vi "BotSpeak_AskDevice.vi"(3 "Bot Settings":T2) -> (1 "Bot Settings out":T2)   [LabVIEW 2012]
uses:
  <userlib>/BotSpeak/VIs/Direct/BotSpeak_Control.ctl
  <vilib>/Platform/browser.llb/Open URL in Default Browser (string).vi
  <userlib>/BotSpeak/VIs/SubVIs/BotSpeak_Globals.vi
panel:
  out "Finished":bool
  in  "View":enum32{"Normal", "Testing"}(tab)
  out "Help":string
  in  "Hardware":u16(ring) items=["Arduino Uno", "BeagleBone Serial", "BeagleBone", "Console Only", "EvalRIO", "Galileo", "Launchpad", "PICAXE 80M", "Raspberry Pi", "Thymio"]
  in  "Done":bool
  in  "Cancel":bool
  in  "Connection":T1(tab)
  in  "IP Address":string(combo)
  in  "VISA":u16(ring) items=["ASRL7  (COM7 - Galileo)", "ASRL4  (COM4 - Intel(R) Active Management Technology - SOL)", "ASRL3  (COM3)"]
  in  "Test":bool
  in  "Goto URL":bool
  out "URL":string
  out "Status":string
  out "firmware":dbl
  in  "Back":bool
  out "List":string[](array[string])
  # "For More Help:"
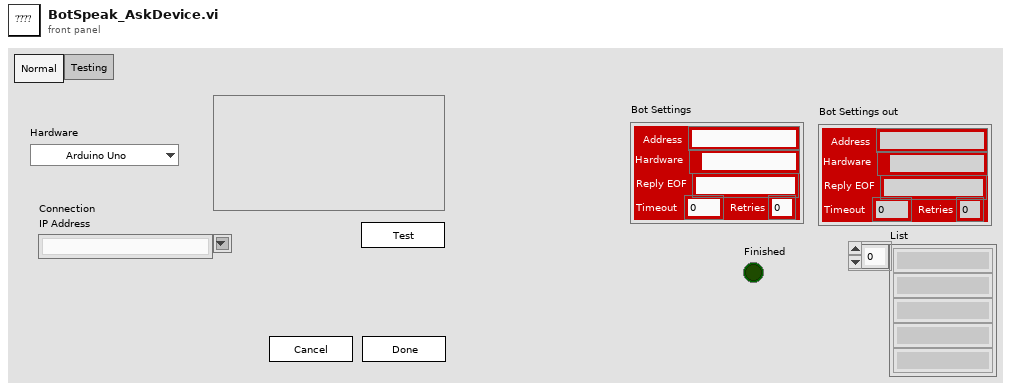
[diagram p1: front panel]
types:
  T1 = enum32{"TCPIP", "Serial", "Undefined", "Console"}
  T2 = typedef "BotSpeak_Control.ctl" = cluster{"Address":string, "Reply EOF":string, "Hardware":path, "Retries":i8, "Timeout":i32}
  T3 = typedef "BotSpeak.HardwareSpecs.ctl" = cluster{"Hardware Name":string, "Hardware URL":string, "ComType":enum16{"Undefined", "Serial", "TCPIP", "Console"}, "TCP Port":i32, "DefaultAddress":string, "Retries":i32, "Translate":enum16{"None", "Tiny", "URAPI"}, "MaxScriptSize":i32, "MaxVarNumber":i32, "StartupWait":i32, "Patience":i32, "Startup Patience":i32, "Hardware Help":string, "Com Protocol":string, "Translator":cluster{"BotSpeak CMD":string, "CMD out":string}[], "Init Code":string, "Variable Format":enum16{"INT", "FLOAT", "FIXED"}}
  T4 = enum16{"Undefined", "Serial", "TCPIP", "Console"}
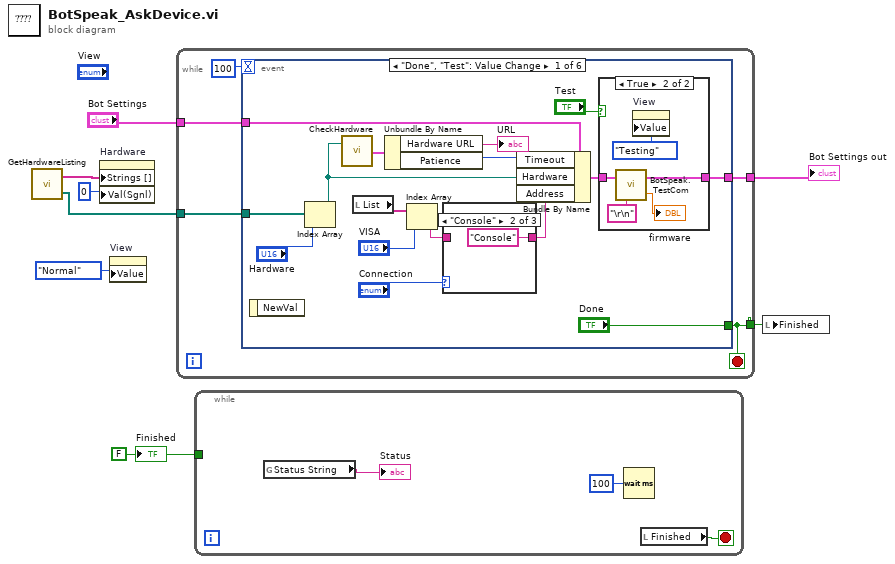
[diagram p0: block diagram]
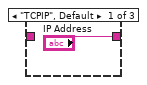
[diagram p2: hidden frame]
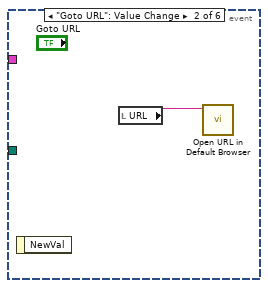
[diagram p5: hidden frame]
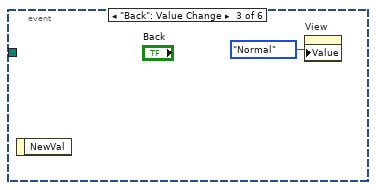
[diagram p6: hidden frame]
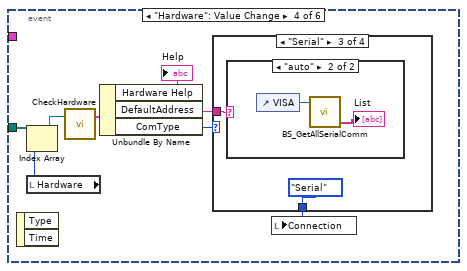
[diagram p7: hidden frame]
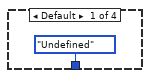
[diagram p8: hidden frame]
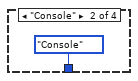
[diagram p9: hidden frame]
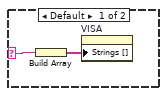
[diagram p10: hidden frame]
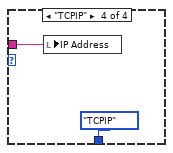
[diagram p11: hidden frame]
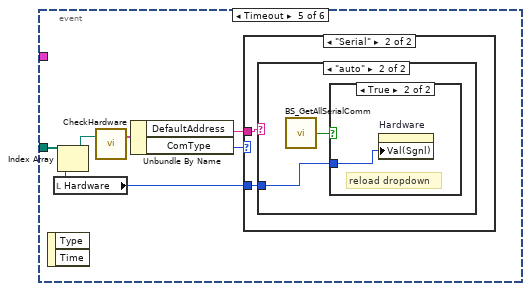
[diagram p12: hidden frame]
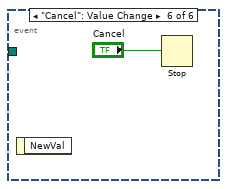
[diagram p16: hidden frame]
diagram:
  w3 = FALSE ("Finished")
  n1 = call <userlib>:"GetHardwareListing.vi"() -> ("Devices"=w1:path[], "Array"=w2:string[])  [unwired: 2 in]
  n2 = property on="Hardware" class="Ring (strict)"("Strings []"=w2, "Val(Sgnl)"=u16 0 ("Value (Signaling)")) -> ()  [unwired: 2 in, 2 out]
  n3 = property on="View" class="TabCtl (strict)"("Value"=enum32{"Normal", "Testing"}."Normal" ("View")) -> ()  [unwired: 2 in, 2 out]
  n4 = while {
    tunnel: [w13] -> w8
    tunnel: w1 -> [w12]
    tunnel: "Bot Settings" -> [w11]
    tunnel: [w9] -> w4
    stop <- w9 stop-if-true
    n5 = event shown="[0] \"Done\", \"Test\": Value Change" {
      selector: _ -> [_ _ _ _ _ _]
      dyn-events: _ -> [_ _ _ _ _ _]
      timeout: 100 -> [_ _ _ _ _ _]
      tunnel: w12 -> [w29 _ _ w48 w64 _]
      tunnel: w11 -> [w27 _ _ _ _ _]
      tunnel: [w19 _ _ _ _ _] -> w13
      tunnel: ["Done" _ _ _ _ _] -> w9
      event "Done", "Test": Value Change {
        n6 = event-data() -> ()  [unwired: 1 in, 1 out]
        n7 = Index Array(array=w29, index="Hardware") -> (element=w18:path)
        n8 = call <userlib>:"CheckHardware.vi"("Hardware"=w18) -> ("HardwareSpecs"=w22:T3)  [unwired: 2 in]
        n9 = local read "List"() -> (w24:string[])
        n10 = Unbundle By Name(w22) -> ("Hardware URL"=→"URL":string, "Patience"=w14:i32)
        n11 = Index Array(array=w24, index="VISA") -> (element=w15:string)
        n12 = case shown="\"Console\"" "Connection" {
          tunnel: ["IP Address" "Console" ("Intf Inst Name") w32] -> w16
          tunnel: w15 -> [_ _ w32]
          frame "TCPIP", Default {
          }
          frame "Console" {
          }
          frame "Serial" {
          }
        }
        n13 = Bundle By Name(cluster=w27, "Timeout"=w14, "Hardware"=w18, "Address"=w16) -> (w20:T2)
        n14 = case shown="True" "Test" {
          tunnel: w20 -> [w33 w35]
          tunnel: [w33 w34] -> w19
          frame False {
          }
          frame True {
            n15 = call <userlib>:"BotSpeak.TestCom.vi"("Termination"="\r\n", "Bot Settings"=w35) -> ("firmware"=→"firmware":dbl, "Bot Settings out"=w34:T2)
            n16 = property on="View" class="TabCtl (strict)"("Value"=enum32{"Normal", "Testing"}."Testing" ("View")) -> ()  [unwired: 2 in, 2 out]
          }
        }
      }
      event "Goto URL": Value Change {
        n17 = event-data() -> ()  [unwired: 1 in, 1 out]
        n18 = local read "URL"() -> (w39:string)
        n19 = call-poly <vilib>:"Open URL in Default Browser.vi"("URL"=w39) -> ()  [unwired: 5 in, 2 out]
      }
      event "Back": Value Change {
        n20 = event-data() -> ()  [unwired: 1 in, 1 out]
        n21 = property on="View" class="TabCtl (strict)"("Value"=enum32{"Normal", "Testing"}."Normal" ("View")) -> ()  [unwired: 2 in, 2 out]
      }
      event "Hardware": Value Change {
        n22 = event-data() -> ()  [unwired: 1 in, 2 out]
        n23 = local read "Hardware"() -> (w42:u16)
        n24 = Index Array(array=w48, index=w42) -> (element=w47:path)
        n25 = call <userlib>:"CheckHardware.vi"("Hardware"=w47) -> ("HardwareSpecs"=w46:T3)  [unwired: 2 in]
        n26 = Unbundle By Name(w46) -> ("Hardware Help"=→"Help":string, "DefaultAddress"=w43:string, "ComType"=w45:T4)
        n27 = case shown="\"Serial\"" w45 {
          tunnel: [enum32{"TCPIP", "Serial", "Undefined"}."Undefined" ("Tabs") T1."Console" ("Connection") enum32{"TCPIP", "Serial", "Undefined"}."Serial" ("Tabs") enum32{"TCPIP", "Serial", "Undefined"}."TCPIP" ("Tabs")] -> w44
          tunnel: w43 -> [_ _ w51 w57]
          frame Default {
          }
          frame "Console" {
          }
          frame "Serial" {
            n28 = case shown="\"auto\"" w51 {
              selector: w51 -> [w54 _]
              frame Default {
                n29 = Build Array(w54) -> (w53:string[])
                n30 = property on="VISA" class="Ring (strict)"("Strings []"=w53) -> ()  [unwired: 2 in, 2 out]
              }
              frame "auto" {
                n31 = control-ref of="VISA"() -> (w56:refnum<vi>)
                n32 = call <userlib>:"BS_GetAllSerialComm.vi"("reference"=w56) -> ("List"=→"List":string[])  [unwired: 1 in, 2 out]
              }
            }
          }
          frame "TCPIP" {
            n33 = local write "IP Address"(w57) -> ()
          }
        }
        n34 = local write "Connection"(w44) -> ()
      }
      event Timeout {
        n35 = event-data() -> ()  [unwired: 1 in, 2 out]
        n36 = local read "Hardware"() -> (w59:u16)
        n37 = Index Array(array=w64, index=w59) -> (element=w63:path)
        n38 = call <userlib>:"CheckHardware.vi"("Hardware"=w63) -> ("HardwareSpecs"=w62:T3)  [unwired: 2 in]
        n39 = Unbundle By Name(w62) -> ("DefaultAddress"=w60:string, "ComType"=w61:T4)
        n40 = case shown="\"Serial\"" w61 {
          tunnel: w60 -> [_ w66]
          tunnel: w59 -> [_ w65]
          frame Default {
          }
          frame "Serial" {
            n41 = case shown="\"auto\"" w66 {
              tunnel: w65 -> [_ w67]
              frame Default {
              }
              frame "auto" {
                n42 = call <userlib>:"BS_GetAllSerialComm.vi"() -> ("new?"=w68:bool)  [unwired: 2 in, 2 out]
                n43 = case shown="True" w68 {
                  tunnel: w67 -> [_ w69]
                  frame False {
                  }
                  frame True {
                    # "reload dropdown"
                    n44 = property on="Hardware" class="Ring (strict)"("Val(Sgnl)"=w69) -> ()  [unwired: 2 in, 2 out]
                  }
                }
              }
            }
          }
        }
      }
      event "Cancel": Value Change {
        n45 = event-data() -> ()  [unwired: 1 in, 1 out]
        n46 = Stop(stop? (T)="Cancel") -> ()
      }
    }
  }
  "Bot Settings out" <- w8
  n47 = while {
    tunnel: w3 -> [_]
    stop <- w71 stop-if-true
    n48 = global read "BotSpeak_Globals.vi" "Status String"() -> (→"Status":string)
    n49 = Wait (ms)(milliseconds to wait=u32 100) -> ()  [unwired: 1 out]
    n50 = local read "Finished"() -> (w71:bool)
  }
  n51 = local write "Finished"(w4) -> ()
  "Finished" <- w3
